vi "d6.1 (hw6).vi"() -> ()   [LabVIEW 2017]
panel:
  out "Array":dbl[](array[numeric])
  in  "Value to Find":dbl
  in  "Array - Numeric":dbl[](array[numeric])
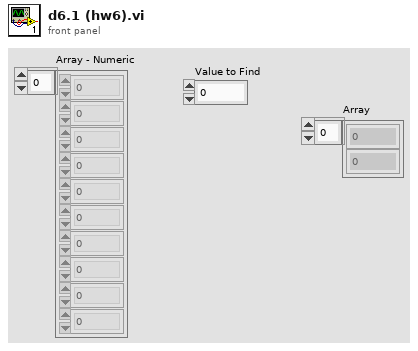
[diagram p1: front panel]
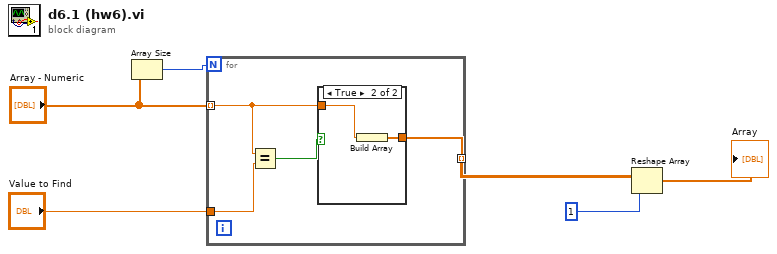
[diagram p0: block diagram]
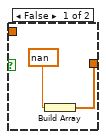
[diagram p2: hidden frame]
diagram:
  n1 = Array Size(array="Array - Numeric") -> (size(s)=w6:i32)
  n2 = for {
    N: w6 -> [_]
    tunnel: "Value to Find" -> [w10]
    tunnel: [w7] -> w1 mode=indexing
    tunnel: "Array - Numeric" -> [w8] mode=indexing
    n3 = Equal?(x=w8, y=w10) -> (x = y?=w9:bool)
    n4 = case shown="True" w9 {
      tunnel: w8 -> [_ w14]
      tunnel: [w12 w13] -> w7
      frame False {
        n5 = Build Array(nan) -> (w12:dbl[])
      }
      frame True {
        n6 = Build Array(w14) -> (w13:dbl[])
      }
    }
  }
  n7 = Reshape Array(w1, 1) -> (→"Array":dbl[])
